vi "CheckButtonPressed.vi"(8 "error in (no error)":errorcluster, 10 "Button":bool) -> (0 "error out":errorcluster, 2 "Pressed?":bool)   [LabVIEW 2013]
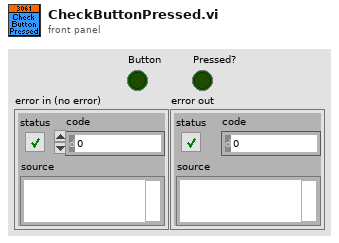
[diagram p1: front panel]
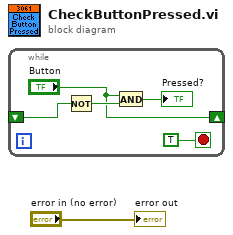
[diagram p0: block diagram]
diagram:
  n1 = while {
    shift-right: ["Button"] -> _
    shift-left: _ -> [w5]
    stop <- TRUE stop-if-true
    n2 = Not(x=w5) -> (.not. x?=w6:bool)
    n3 = And(x="Button", y=w6) -> (x .and. y?=→"Pressed?":bool)
  }
  "error out" <- "error in (no error)"
